vi "Send Single Trigger.vi"(8 "error in (no error)":errorcluster, 11 "VNA-PNA in":refnum<class "VNA-PNA.lvclass">) -> (0 "error out":errorcluster, 3 "VNA-PNA out":refnum<class "VNA-PNA.lvclass">)   [LabVIEW 2020, in "VNA-PNA.lvclass"]
doc: "Sent a single trigger for the VNA. It uses the OPC command to wait until completion.\nIt will use (sweeptime * N average * N ports) for the VISA timeout."
uses:
  VNA-PNA.lvclass
  C:/Sandbox/Git_Sandbox/WiSpry Test Framework source code (LV20)/WiSpry Test Framework/Instruments/Vector Network Analyzer/Vector Network Analyzer.lvclass
  C:/Sandbox/Git_Sandbox/WiSpry Test Framework source code (LV20)/WiSpry Test Framework/Instruments/Instrument.lvclass
  Vector Network Analyzer.lvclass/Vector Network Analyzer.ctl
  Instrument.lvclass/Instrument.ctl
  Vector Network Analyzer.lvclass
  Instrument.lvclass
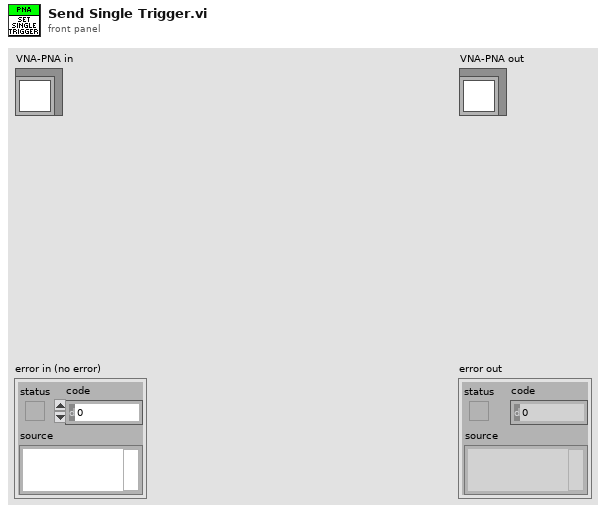
[diagram p1: front panel]
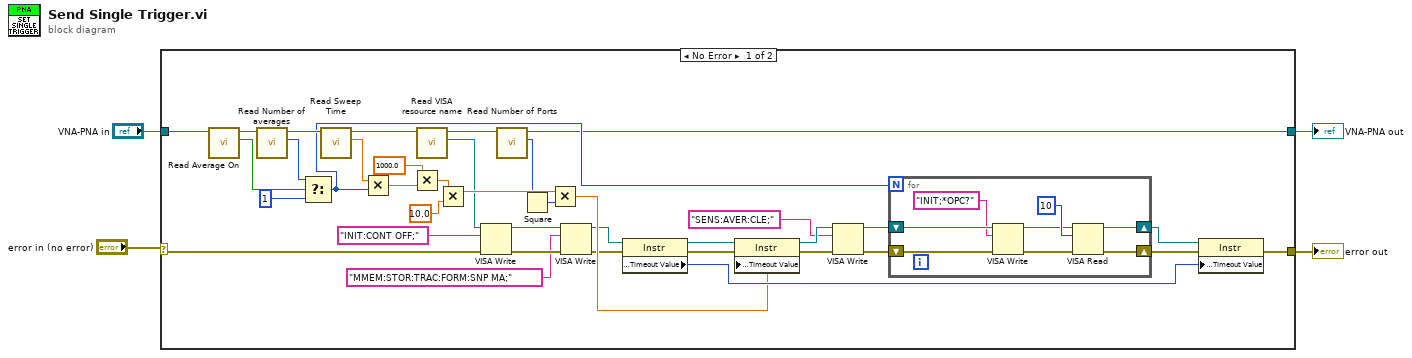
[diagram p0: block diagram]
diagram:
  n1 = case shown="No Error" "error in (no error)" {
    selector: "error in (no error)" -> [w18 w52]
    tunnel: "VNA-PNA in" -> [w42 w51]
    tunnel: [w12 w51] -> w2
    tunnel: [w22 w52] -> w1
    frame No Error {
      n2 = call "Read Average On.vi"("Vector Network Analyzer in"=w42) -> ("Average On"=w38:bool, "Vector Network Analyzer out"=w41:refnum<class "VNA-PNA.lvclass">)  [unwired: 9 in]
      n3 = call "Read Number of averages.vi"("Vector Network Analyzer in"=w41) -> ("Number of averages"=w39:i32, "Vector Network Analyzer out"=w40:refnum<class "VNA-PNA.lvclass">)  [unwired: 9 in]
      n4 = Select(t=w39, s=w38, f=1) -> (s? t:f=w15:i32)
      n5 = call "Read Sweep Time.vi"("Vector Network Analyzer in"=w40) -> ("Sweep Time"=w36:dbl, "Vector Network Analyzer out"=w35:refnum<class "VNA-PNA.lvclass">)  [unwired: 9 in]
      n6 = Multiply(x=w36, y=w15) -> (x*y=w32:dbl)
      n7 = Multiply(x=1000.0, y=w32) -> (x*y=w31:dbl)
      n8 = call "Read VISA resource name.vi"("Instrument in"=w35) -> ("VISA resource name"=w19:refnum<visa-resource-name>, "Instrument out"=w13:refnum<class "VNA-PNA.lvclass">)  [unwired: 9 in]
      n9 = Multiply(x=w31, y=10.0) -> (x*y=w27:dbl)
      n10 = VISA Write(VISA resource name=w19, write buffer="INIT:CONT OFF;", error in (no error)=w18) -> (VISA resource name out=w7:refnum<visa-resource-name>, error out=w6:errorcluster)  [unwired: 1 out]
      n11 = call "Read Number of Ports.vi"("Vector Network Analyzer in"=w13) -> ("Number of Ports"=w10:i32, "Vector Network Analyzer out"=w12:refnum<class "VNA-PNA.lvclass">)  [unwired: 9 in]
      n12 = Square(x=w10) -> (x^2=w11:i32)
      n13 = Multiply(x=w27, y=w11) -> (x*y=w14:dbl)
      n14 = VISA Write(VISA resource name=w7, write buffer="MMEM:STOR:TRAC:FORM:SNP MA;", error in (no error)=w6) -> (VISA resource name out=w8:refnum<visa-resource-name>, error out=w9:errorcluster)  [unwired: 1 out]
      n15 = property class="Instr"(reference=w8, error in=w9) -> (reference out=w34:refnum<visa-resource-name>, error out=w33:errorcluster, "General Settings:Timeout Value"=w24:u32)
      n16 = property class="Instr"(reference=w34, error in=w33, "General Settings:Timeout Value"=w14) -> (reference out=w29:refnum<visa-resource-name>, error out=w28:errorcluster)
      n17 = VISA Write(VISA resource name=w29, write buffer="SENS:AVER:CLE;", error in (no error)=w28) -> (VISA resource name out=w20:refnum<visa-resource-name>, error out=w21:errorcluster)  [unwired: 1 out]
      n18 = for {
        N: w15 -> [_]
        shift-right: [w49] -> w23
        shift-left: w21 -> [w47]
        shift-right: [w50] -> w25
        shift-left: w20 -> [w46]
        n19 = VISA Write(VISA resource name=w46, write buffer="INIT;*OPC?", error in (no error)=w47) -> (VISA resource name out=w45:refnum<visa-resource-name>, error out=w44:errorcluster)  [unwired: 1 out]
        n20 = VISA Read(VISA resource name=w45, byte count=u32 10, error in (no error)=w44) -> (VISA resource name out=w50:refnum<visa-resource-name>, error out=w49:errorcluster)  [unwired: 2 out]
      }
      n21 = property class="Instr"(reference=w25, error in=w23, "General Settings:Timeout Value"=w24) -> (error out=w22:errorcluster)  [unwired: 1 out]
    }
    frame Error {
    }
  }
  "error out" <- w1
  "VNA-PNA out" <- w2
